vi "사용자 컨트롤.vi"   [LabVIEW 2014]
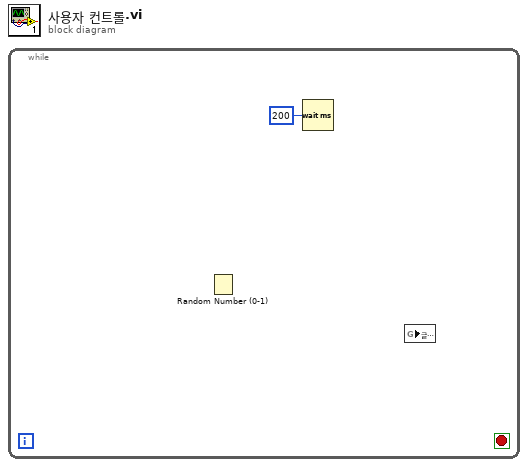
[diagram p0: block diagram]
diagram:
  n1 = while {
    stop <- _ stop-if-true
    n2 = Random Number (0-1)() -> ()  [unwired: 1 out]
    n3 = Wait (ms)(milliseconds to wait=u32 200 ("대기 시간(ms)")) -> ()  [unwired: 1 out]
    n4 = global read "글로벌 1.vi" item#-1() -> ()  [unwired: 1 in]
  }
